vi "Perform Action.vi"(8 "error in":errorcluster, 10 "Input":variant, 11 "AI DAQmx Cont CFG in":refnum<class "AI Current DAQmx Cont CFG.lvclass">) -> (0 "error out":errorcluster, 2 "Output":variant, 3 "AI DAQmx Cont CFG out":refnum<class "AI Current DAQmx Cont CFG.lvclass">)   [LabVIEW 2024, in "AI Current DAQmx Cont CFG.lvclass"]
uses:
  AI Current DAQmx Cont CFG.lvclass
  AI Current DAQmx Cont CFG.lvclass/AI Current DAQmx Cont CFG.ctl
  DAQmx Base CFG/DAQmx Base CFG.lvclass
  Buffers/BufferLastReadingsDBL/BufferLastReadsDBL.lvclass
  <vilib>/DAQmx/read.llb/DAQmx Read (Analog 2D DBL NChan NSamp).vi
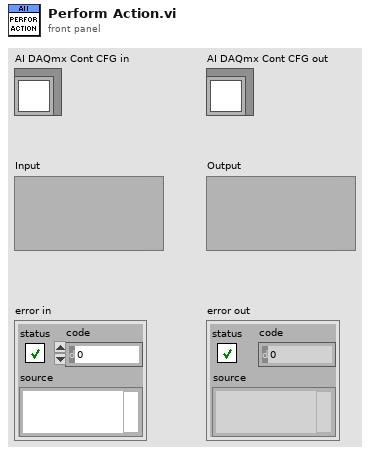
[diagram p1: front panel]
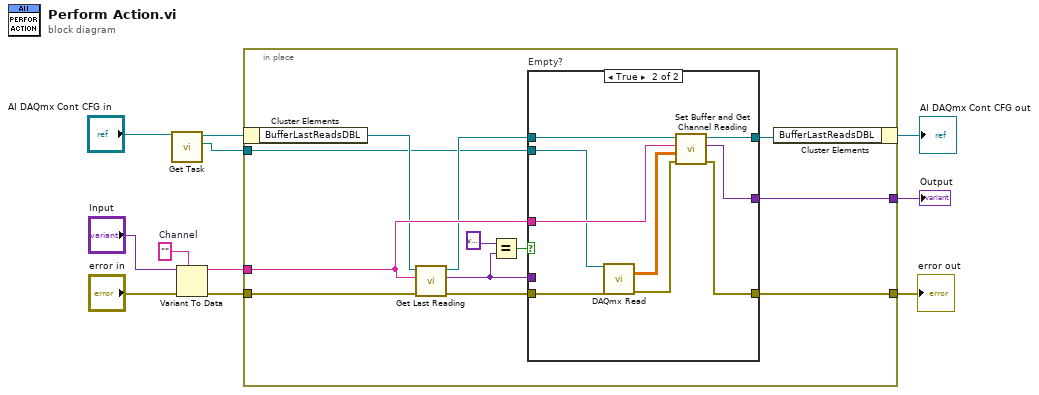
[diagram p0: block diagram]
diagram:
  w7 = ""  # Channel
  n1 = call "Get Task.vi"("DAQmx Base CFG in"="AI DAQmx Cont CFG in") -> ("Task"=w4:refnum<k21>, "DAQmx Base CFG out"=w2:refnum<class "AI Current DAQmx Cont CFG.lvclass">)  [unwired: 9 in]
  n2 = Variant To Data(error in="error in", type=w7, Variant="Input") -> (data=w5:string, error out=w6:errorcluster)
  n3 = in-place {
    in-place-border: [w23] -> w9
    in-place-border: [w22] -> w8
    in-place-border: w6 -> [w21]
    in-place-border: w5 -> [w20]
    in-place-border: w4 -> [w13]
    n4 = in-place-cluster #1(w2) -> ("BufferLastReadsDBL"=w14:refnum<class "BufferLastReadsDBL.lvclass">)
    n5 = call "Get Last Reading.vi"("error in"=w21, "Channel"=w20, "BufferLastReadingsDBL in"=w14) -> ("error out"=w19:errorcluster, "Last Read"=w16:variant, "BufferLastReadingsDBL out"=w18:refnum<class "BufferLastReadsDBL.lvclass">)  [unwired: 6 in]
    n6 = Equal?(x=variant, y=w16) -> (x = y?=w17:bool)
    n7 = case "Empty?" shown="True" w17 {
      tunnel: [w25 w33] -> w23
      tunnel: w18 -> [w24 w35]
      tunnel: [w26 w30] -> w22
      tunnel: w16 -> [w26 _]
      tunnel: w19 -> [w25 w32]
      tunnel: w20 -> [_ w31]
      tunnel: w13 -> [_ w28]
      tunnel: [w24 w27] -> w12
      frame False {
      }
      frame True {
        n8 = call-poly <vilib>:"DAQmx Read.vi"("task/channels in"=w28, "error in"=w32) -> ("data"=w34:dbl[][], "error out"=w29:errorcluster)  [unwired: 11 in, 1 out]
        n9 = call "Set Buffer and Get Channel Reading.vi"("error in"=w29, "Readings"=w34, "Channel Ident"=w31, "BufferLastReadingsDBL in"=w35) -> ("error out"=w33:errorcluster, "Last Read"=w30:variant, "BufferLastReadingsDBL out"=w27:refnum<class "BufferLastReadsDBL.lvclass">)  [unwired: 5 in]
      }
    }
    n10 = in-place-cluster #1("BufferLastReadsDBL"=w12) -> (→"AI DAQmx Cont CFG out":refnum<class "AI Current DAQmx Cont CFG.lvclass">)
  }
  "error out" <- w9
  "Output" <- w8
